vi "Task_05.vi"() -> ()   [LabVIEW 2018]
uses:
  <vilib>/Utility/file.llb/Read Delimited Spreadsheet (string).vi
  <vilib>/Utility/file.llb/Read Delimited Spreadsheet (DBL).vi
panel:
  in  "Stop Button":bool
  in  "Начать":bool
  in  "Cluster":T1 caption="Отображение параметров"
  out "Waveform Chart":waveform(dbl)[](graph)
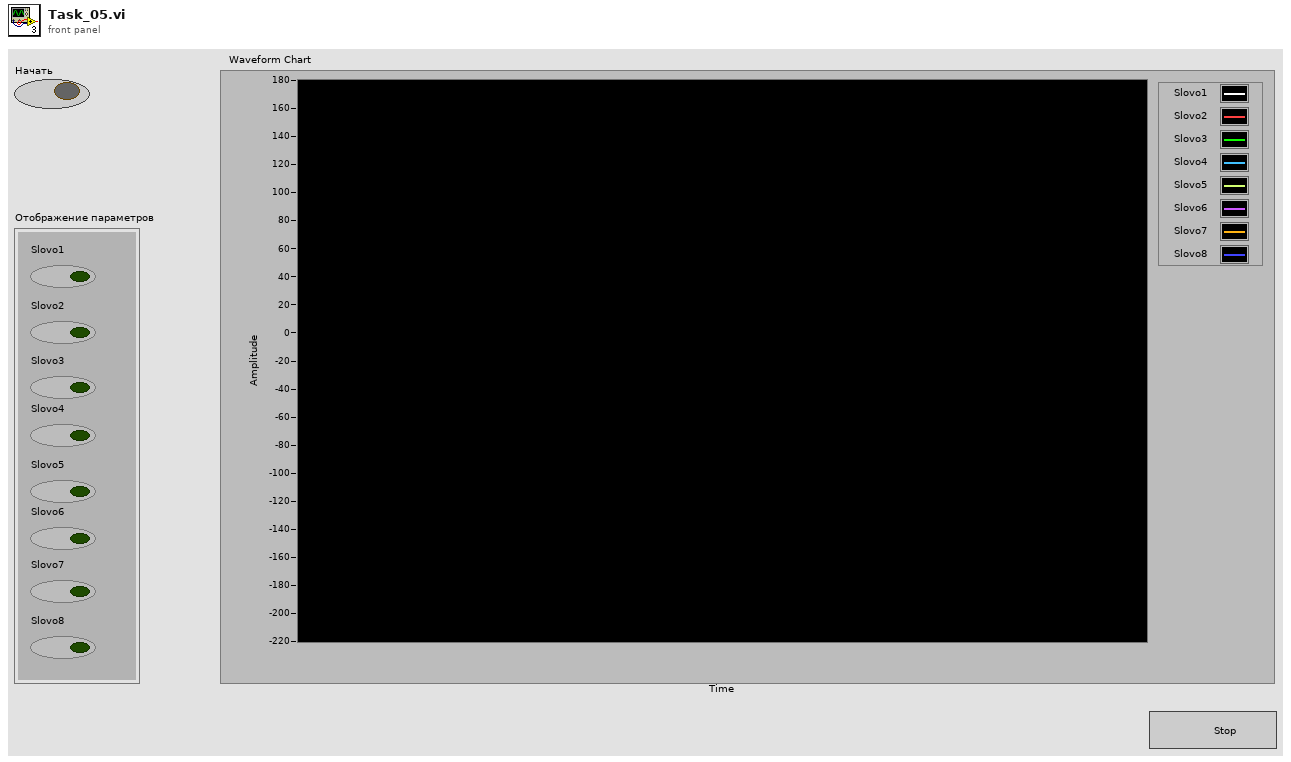
[diagram p1: front panel]
types:
  T1 = cluster{"Slovo1":bool, "Slovo2":bool, "Slovo3":bool, "Slovo4":bool, "Slovo5":bool, "Slovo6":bool, "Slovo7":bool, "Slovo8":bool}
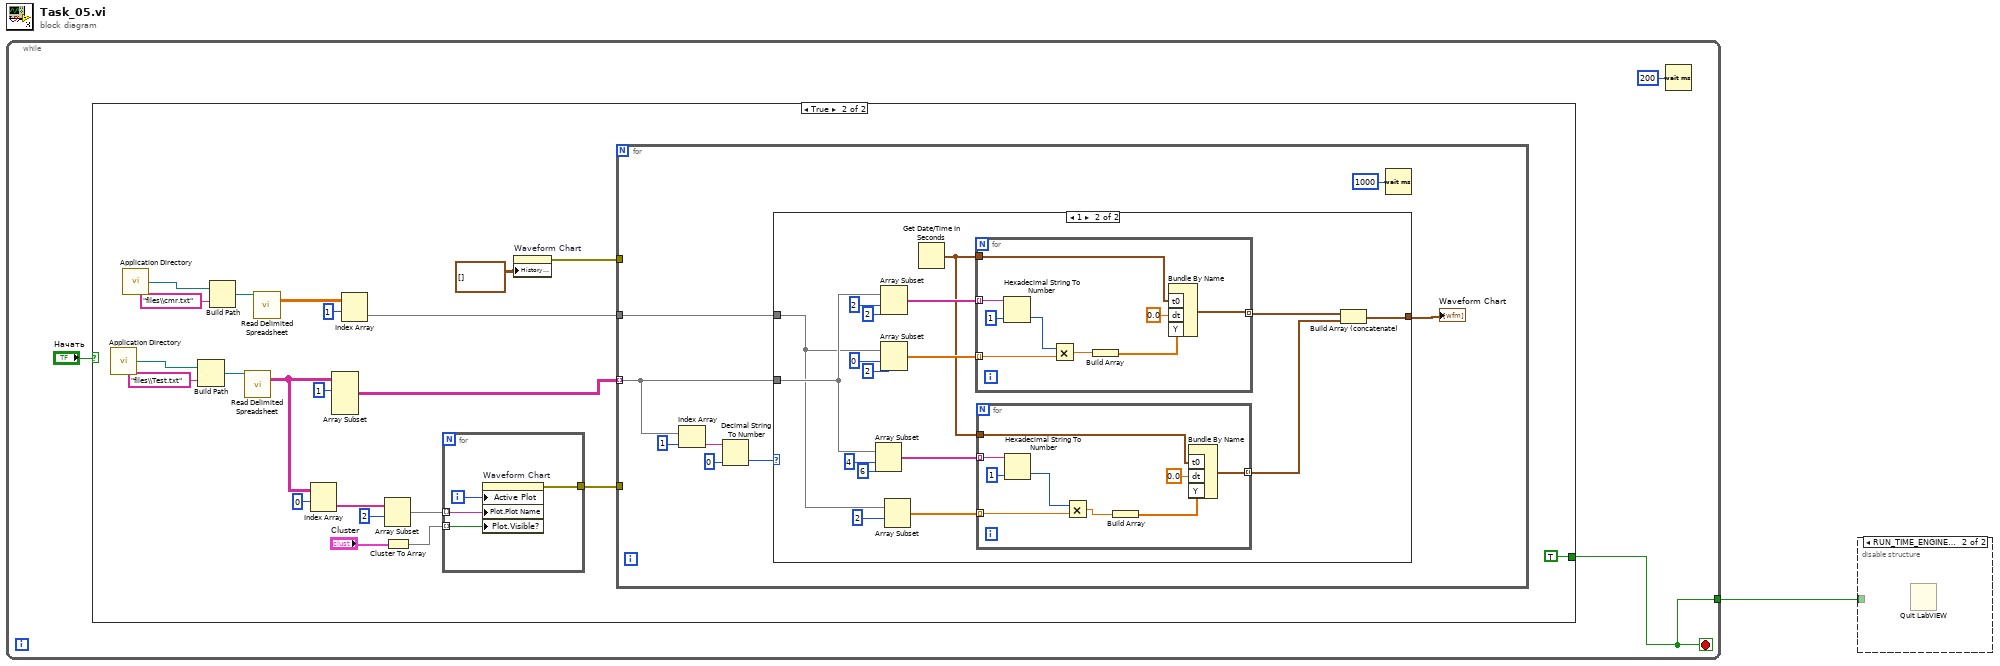
[diagram p0: block diagram]
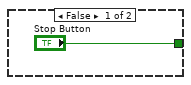
[diagram p3: hidden frame]
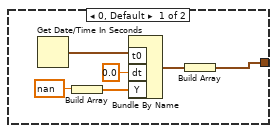
[diagram p4: hidden frame]
diagram:
  n1 = while {
    tunnel: [w2] -> w1
    stop <- w2 stop-if-true
    n2 = case shown="True" "Начать" {
      tunnel: ["Stop Button" TRUE ("Stop Button")] -> w2
      frame False {
      }
      frame True {
        n3 = call <vilib>:"Application Directory.vi"() -> ("Application Directory"=w27:path)
        n4 = call <vilib>:"Application Directory.vi"() -> ("Application Directory"=w19:path)
        n5 = Build Path(base path=w27, name or relative path="files\\Test.txt") -> (appended path=w25:path)
        n6 = Build Path(base path=w19, name or relative path="files\\cmr.txt") -> (appended path=w18:path)
        n7 = call-poly <vilib>:"Read Delimited Spreadsheet.vi"("file path (dialog if empty)"=w25) -> ("all rows"=w14:string[][])  [unwired: 9 in, 5 out]
        n8 = call-poly <vilib>:"Read Delimited Spreadsheet.vi"("file path (dialog if empty)"=w18) -> ("all rows"=w17:dbl[][])  [unwired: 9 in, 5 out]
        n9 = Index Array(array=w14, index (row)=0) -> (element=w23:string[])  [unwired: 1 in]
        n10 = Array Subset(array=w14, index (row)=1 ("index")) -> (w13:string[][])  [unwired: 3 in]
        n11 = Index Array(array=w17, index (row)=1) -> (element=w15:dbl[])  [unwired: 1 in]
        n12 = Array Subset(array=w23, index=2) -> (w21:string[])  [unwired: 1 in]
        n13 = Cluster To Array(cluster="Cluster") -> (array=w10:bool[])
        n14 = for {
          tunnel: w21 -> [w80] mode=indexing
          tunnel: w10 -> [w78] mode=indexing
          tunnel: [w77] -> w9
          i -> [w79]
          n15 = property on="Waveform Chart" class="WFChart (strict)"("Active Plot"=w79, "Plot.Plot Name"=w80, "Plot.Visible?"=w78) -> (error out=w77:errorcluster)  [unwired: 2 in, 1 out]
        }
        n16 = property on="Waveform Chart" class="WFChart (strict)"("History Data"=waveform(dbl)[][] []) -> (error out=w7:errorcluster)  [unwired: 2 in, 1 out]
        n17 = for {
          tunnel: w13 -> [w31] mode=indexing
          tunnel: w15 -> [w30]
          tunnel: w9 -> [_]
          tunnel: w7 -> [_]
          n18 = Index Array(array=w31, index=1) -> (element=w34:string)
          n19 = Decimal String To Number(string=w34, default (0L)=u8 0 ("default (0 I32)")) -> (number=w32:u8)  [unwired: 1 in, 1 out]
          n20 = case shown="1" w32 {
            tunnel: w31 -> [_ w50]
            tunnel: w30 -> [_ w48]
            tunnel: [w36 w42] -> w28
            frame 0, Default {
              n21 = Get Date/Time In Seconds() -> (seconds since 1Jan1904=w41:timestamp)
              n22 = Build Array(nan) -> (w39:dbl[])
              n23 = Bundle By Name("t0"=w41, "dt"=0.0, "Y"=w39) -> (w37:waveform(dbl))  [unwired: 1 in]
              n24 = Build Array(w37) -> (w36:waveform(dbl)[])
            }
            frame 1 {
              n25 = Array Subset(array=w50, index=4, length=6) -> (w47:string[])
              n26 = Array Subset(array=w50, index=2, length=2) -> (w56:string[])
              n27 = Array Subset(array=w48, index=0, length=2) -> (w51:dbl[])
              n28 = Array Subset(array=w48, index=2) -> (w46:dbl[])  [unwired: 1 in]
              n29 = Get Date/Time In Seconds() -> (seconds since 1Jan1904=w45:timestamp)
              n30 = for {
                tunnel: w56 -> [w75] mode=indexing
                tunnel: w51 -> [w73] mode=indexing
                tunnel: w45 -> [w69]
                tunnel: [w68] -> w44 mode=indexing
                n31 = Hexadecimal String To Number(string=w75, default (0uL)=u16 1 ("default (0 U32)")) -> (number=w74:u16)  [unwired: 1 in, 1 out]
                n32 = Multiply(x=w74, y=w73) -> (x*y=w72:dbl)
                n33 = Build Array(w72) -> (w71:dbl[])
                n34 = Bundle By Name("t0"=w69, "dt"=0.0, "Y"=w71) -> (w68:waveform(dbl))  [unwired: 1 in]
              }
              n35 = for {
                tunnel: w47 -> [w66] mode=indexing
                tunnel: w46 -> [w64] mode=indexing
                tunnel: w45 -> [w60]
                tunnel: [w59] -> w43 mode=indexing
                n36 = Hexadecimal String To Number(string=w66, default (0uL)=i16 1 ("default (0 U32)")) -> (number=w65:i16)  [unwired: 1 in, 1 out]
                n37 = Multiply(x=w65, y=w64) -> (x*y=w61:dbl)
                n38 = Build Array(w61) -> (w62:dbl[])
                n39 = Bundle By Name("t0"=w60, "dt"=0.0, "Y"=w62) -> (w59:waveform(dbl))  [unwired: 1 in]
              }
              n40 = Build Array (concatenate)(w44, w43) -> (w42:waveform(dbl)[])
            }
          }
          "Waveform Chart" <- w28
          n41 = Wait (ms)(milliseconds to wait=u32 1000) -> ()  [unwired: 1 out]
        }
      }
    }
    n42 = Wait (ms)(milliseconds to wait=u32 200) -> ()  [unwired: 1 out]
  }
  n43 = disable-structure shown="RUN_TIME_ENGINE==True" {
    disable-tunnel: w1 -> [_ _]
    frame condition #0 (active) {
    }
    frame condition #1 {
      n44 = Quit LabVIEW() -> ()  [unwired: 1 in]
    }
  }
